vi "RT Target, Main.vi"() -> ()   [LabVIEW 2019]
uses:
  <vilib>/Platform/TimedLoop/XDataNode/timing_clust.ctl
  <vilib>/Platform/TimedLoop/XDataNode/nitl_modes.ctl
  <vilib>/Platform/TimedLoop/XDataNode/wakeup.ctl
  <vilib>/FPGAPlugInAG/cRIO-9114/niLvFpga_Open_cRIO-9114.vi
  <vilib>/rvi/interface/common/dynamic/niFpgaDynamicAddResources.vi
  <vilib>/FPGAPlugInAG/Dynamic/niLvFpga_Run_Dynamic.vi
  <vilib>/Utility/error.llb/Error Cluster From Error Code.vi
  <vilib>/rvi/errors/niLvFpgaAdjustHostInterfaceError.vi
  <vilib>/FPGAPlugInAG/Dynamic/niLvFpga_Close_Dynamic.vi
  <vilib>/platform/TimedLoop/XDataNode/XDataNode.xnode
  <vilib>/rvi/interface/nirviOpenFPGA/nirviOpenFPGA.xnode
  FPGA Bitfiles/StepResponse_FPGATarget_FPGATarget,AI0&A_vmHLnBOGIyo.lvbitx
  <vilib>/rvi/interface/nirviMethod/nirviMethod.xnode
  <vilib>/rvi/interface/nirviCloseFPGA/nirviCloseFPGA.xnode
  <vilib>/Platform/TimedLoop/XDataNode/XDNodeRunTimeDep.lvlib
  <vilib>/FPGAPlugInAG/Dynamic/niLvFpga_ReadFifo_Dynamic.vi
  <vilib>/rvi/errors/niLvFpgaMergeErrorWithErrorCode.vi
panel:
  in  "stop":bool
  out "Data Chart":dbl[](graph)
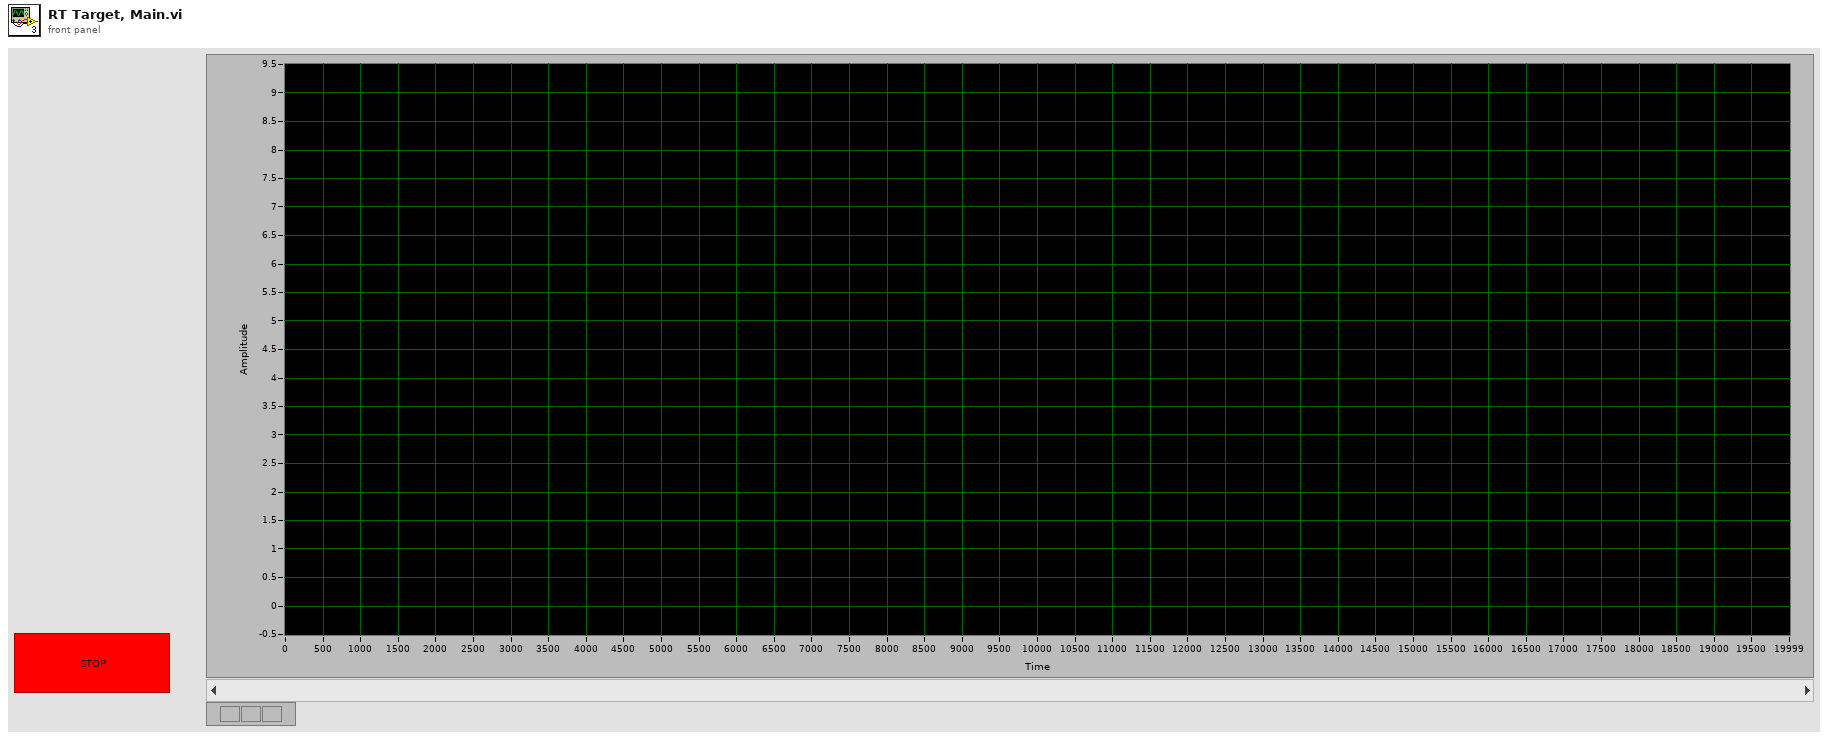
[diagram p1: front panel]
types:
  T1 = typedef "XDNodeRunTimeDep.lvlib/timing_clust.ctl" = cluster{"Expected End [f-1]":u64, "Actual End [f-1]":u64, "Finished Late? [f-1]":bool, "Expected End [i-1]":u64, "Actual End [i-1]":u64, "Finished Late? [i-1]":bool, "Expected Start [i]":u64, "Actual Start [i]":u64, "Expected Start [f]":u64, "Actual Start [f]":u64, "Source Name":string, "Structure Name":string, "Period":i64, "Deadline":i64, "Offset":i64, "Start":i64, "Priority":i32, "Timeout":i32, "Mode":T2, "Wakeup Reason":T3, "Error":errorcluster, "Source Type":string, "Secondary Source Type":string, "Global End Time":u64, "Global Start Time":u64, "Frame Duration":u64, "Iteration Duration":u64, "Assigned CPU":i32, "I/O Scan Engine Mode":u32}
  T2 = typedef "XDNodeRunTimeDep.lvlib/nitl_modes.ctl" = enum32{"No Change", "Process missed periods, maintain original phase", "Discard missed periods, maintain original phase", "Process missed periods, ignore original phase", "Discard missed periods, ignore original phase"}
  T3 = typedef "XDNodeRunTimeDep.lvlib/wakeup.ctl" = enum32{"Normal", "Aborted", "Asynchronous wakeup", "Timing source error", "Timed loop error", "Timeout"}
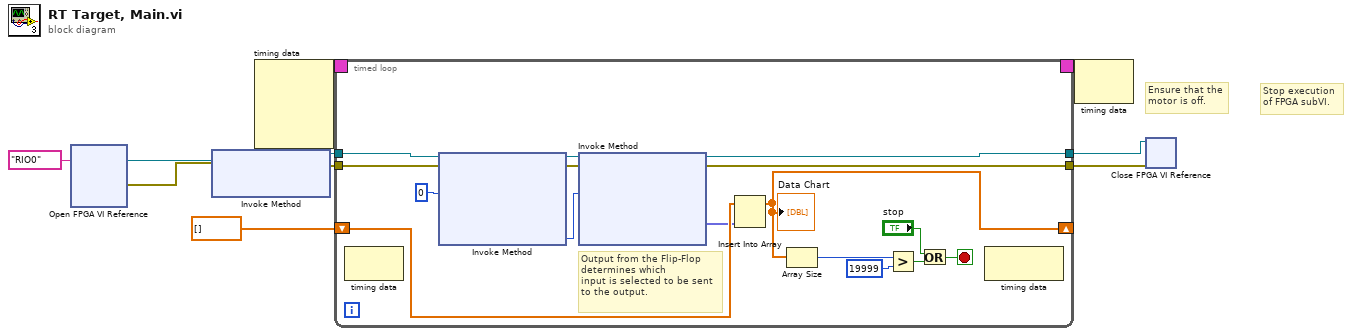
[diagram p0: block diagram]
diagram:
  # "Stop execution\nof FPGA subVI."
  # "Ensure that the\nmotor is off."
  n1 = xnode "Open FPGA VI Reference"("resource name"=tag "RIO0") -> ("FPGA VI Reference Out"=w2:refnum<k20>, "error out"=w1:errorcluster)  [unwired: 1 in]
  n2 = xnode "Invoke Method"("FPGA VI Reference In"=w2, "error in"=w1) -> ("FPGA VI Reference Out"=w7:refnum<k20>, "error out"=w6:errorcluster)  [unwired: 1 in]
  n3 = node-c288() -> (w10:T1)  [unwired: 4 in]
  n4 = timed-loop {
    timing: w10 -> [_]
    timing-out: [_] -> w9
    tunnel: [w24] -> w8
    tunnel: w7 -> [w25]
    tunnel: w6 -> [w20]
    tunnel: [w18] -> w5
    shift-right: [w11] -> _
    shift-left: dbl[] [] -> [w17]
    stop <- w12 stop-if-true
    # "Output from the Flip-Flop\ndetermines which\ninput is selected to be sent\nto the output."
    n5 = node-c288() -> ()  [unwired: 1 in, 1 out]
    n6 = xnode "Invoke Method"("FPGA VI Reference In"=w25, "error in"=w20, "Number of Elements"=u32 0) -> ("FPGA VI Reference Out"=w23:refnum<k20>, "error out"=w19:errorcluster, "Elements Remaining"=w22:u32)  [unwired: 1 in, 1 out]
    n7 = xnode "Invoke Method"("FPGA VI Reference In"=w23, "error in"=w19, "Number of Elements"=w22) -> ("FPGA VI Reference Out"=w24:refnum<k20>, "error out"=w18:errorcluster, "Data"=w16:fxp<+/-,20,5>[])  [unwired: 1 in, 1 out]
    n8 = Insert Into Array(array=w17, new element=w16) -> (w11:dbl[])  [unwired: 1 in]
    "Data Chart" <- w11
    n9 = Array Size(array=w11) -> (size(s)=w15:i32)
    n10 = Greater?(x=w15, y=19999) -> (0:w13:bool)
    n11 = Or(x="stop", y=w13) -> (x .or. y?=w12:bool)
    n12 = node-c288() -> ()  [unwired: 1 in, 1 out]
  }
  n13 = node-c288(w9) -> ()  [unwired: 1 out]
  n14 = xnode "Close FPGA VI Reference"("FPGA VI Reference In"=w8, "error in"=w5) -> ()  [unwired: 1 out]
